vi "Complex Multiply.vi"(4 "path in":path, 5 "input":cluster{"re":dbl, "im":dbl}) -> (1 "function return":i32, 2 "output":dbl)   [LabVIEW 2018, in "Labview_to_DLL.lvlib"]
doc: "extern \"C\" __declspec(dllexport) int ComplexMultiply(cmplx64* input, double* output);"
uses:
  Labview_to_DLL.lvlib
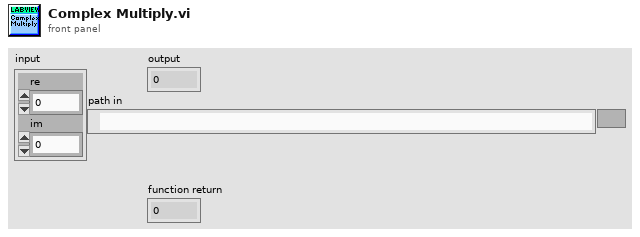
[diagram p1: front panel]
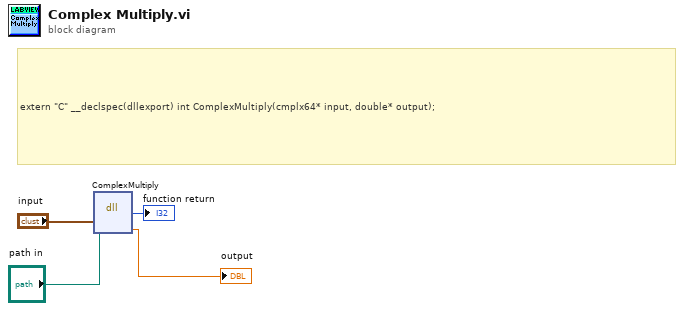
[diagram p0: block diagram]
diagram:
  # "extern \"C\" __declspec(dllexport) int ComplexMultiply(cmplx64* input, double* output);"
  n1 = dll-call lib="C:/Users/celit/Documents/GitHub/Labview_Python_DLL_Call/vs/Debug/Labview_to_DLL.*" fn="ComplexMultiply"(path in="path in", "input"="input") -> ("return type"=→"function return":i32, "output"=→"output":dbl)  [unwired: 4 in, 2 out]
